vi "myRIO_BRig_FPGA_v3,61__PortC.vi"() -> ()   [LabVIEW 2014]
uses:
  <vilib>/rvi/Emulation/niFpgaGetClockAttributes.vi
  <vilib>/rvi/Emulation/niFpgaSctlEmulationGetInTimedLoop.vi
  <vilib>/rvi/Emulation/niFpgaEmulationReportErrorSimple.vi
  <vilib>/rvi/eio/common/nirviEmuTemplateMethod_errors.vi
  <vilib>/rvi/Emulation/niFpgaCriticalErrorInLSC.vi
  <vilib>/eio/EIONode/EIONode.xnode
panel:
  in  "laser2_selRew_Ntotal":u32=100
  in  "laser2selWro_Ntotal":u32=100
  in  "laser2_selRew_Ndelay":u32
  in  "laser2_selWro_Ndelay":u32
  in  "laser2_Npeak":u32=100
  in  "laser2_Nvalley":u32=100
  in  "laser2_Nshutter":u32=100
  in  "laser2_On":bool
  in  "laser2_Event":bool
  out "AnaIn_1":i16
  out "AnaIn_0":i16
  out "count_timeTrial":u32
  in  "timeTrial":bool
  in  "k1__counter_per_ms":u16=100 min=100 max=40000 step=1
  in  "laser1_Nshutter":u32=100
  in  "AnaOut_0":i16
  in  "laser1_Nvalley":u32=100
  in  "laser1_Npeak":u32=100
  in  "laser1_Event":bool
  in  "laser1_selWro_Ntotal":u32=100
  in  "laser1_selWro_Ndelay":u32
  in  "laser1_selRew_Ntotal":u32=100
  in  "laser1_selRew_Ndelay":u32
  in  "laserResponse_reward_LED":bool
  in  "laserResponse_wrong_LED":bool
  out "SelectWrong":bool
  out "SelectReward":bool
  in  "laserResponse_wrong":bool
  in  "laserResponse_reward":bool
  in  "Left(F)_or_Right(T)":bool
  in  "ignoreWrong":bool
  in  "SelectionState":bool
  in  "laser1_On":bool
  in  "FPGA_Stop":bool
  in  "audioTrigger_L":bool
  in  "audioTrigger_R":bool
  in  "audioFreq_L_kHz":u8=14 min=1 max=14 step=1
  in  "audioAmp_L":u16=1 min=1 max=32767 step=1
  in  "audioFreq_R_kHz":u8=14 min=1 max=14 step=1
  in  "audioAmp_R":u16=1 min=1 max=32767 step=1
  in  "A3_SL":bool
  in  "A1_SR":bool
  in  "Counts_Reset":bool
  out "A4_LickR":u32
  out "A2_LickL":u32
  in  "A6_Act":bool
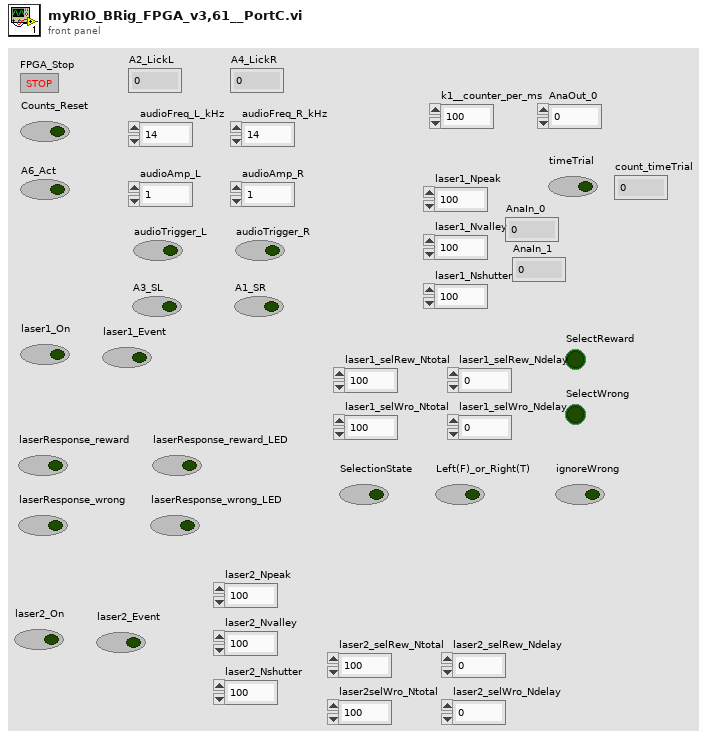
[diagram p1: front panel]
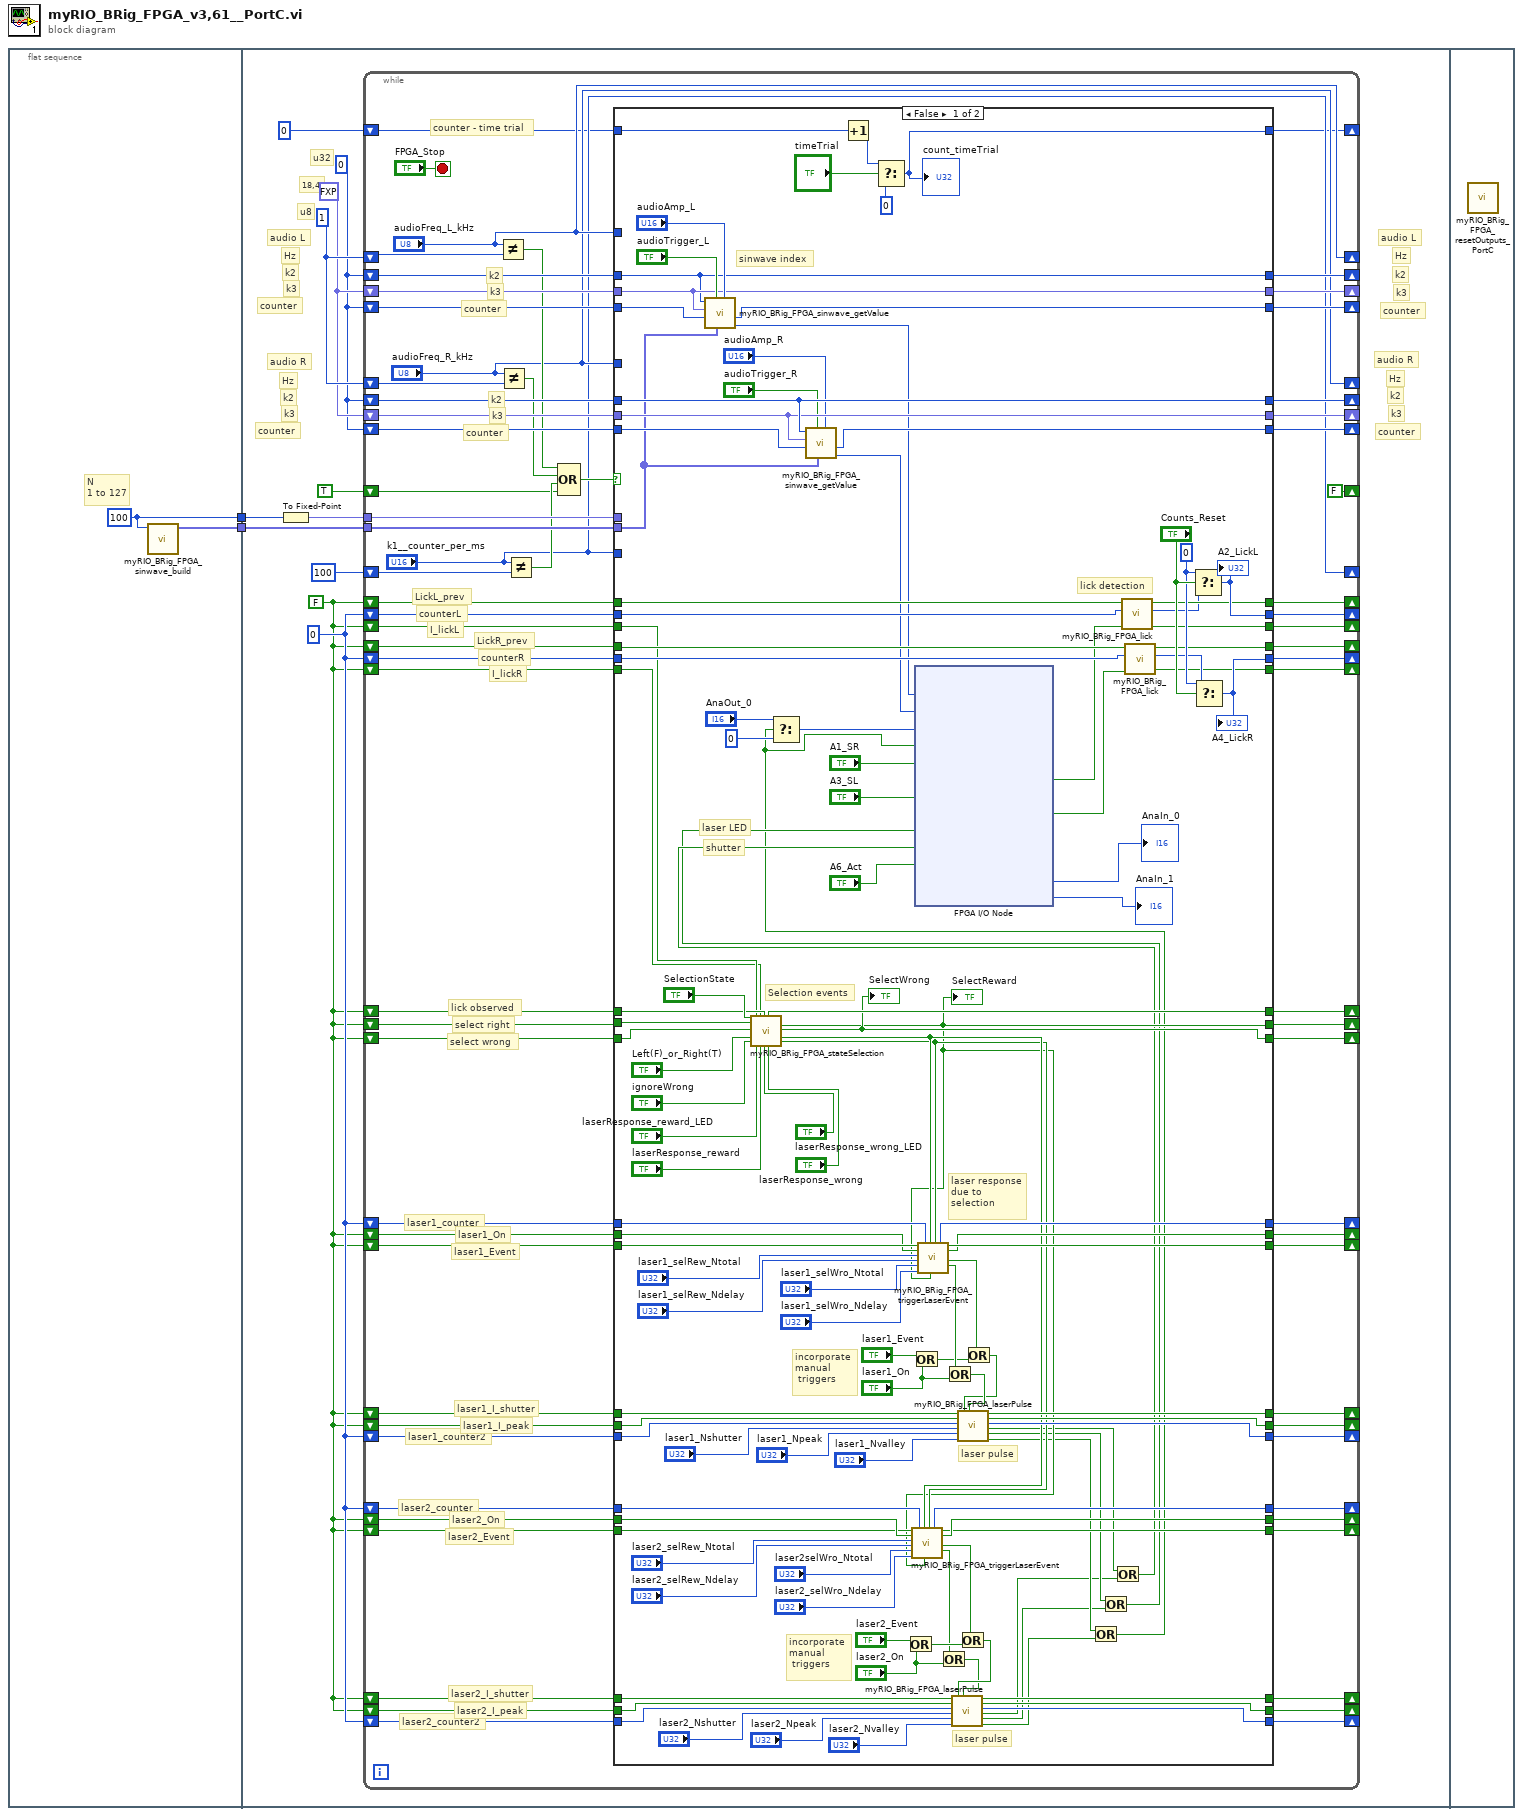
[diagram p0: block diagram]
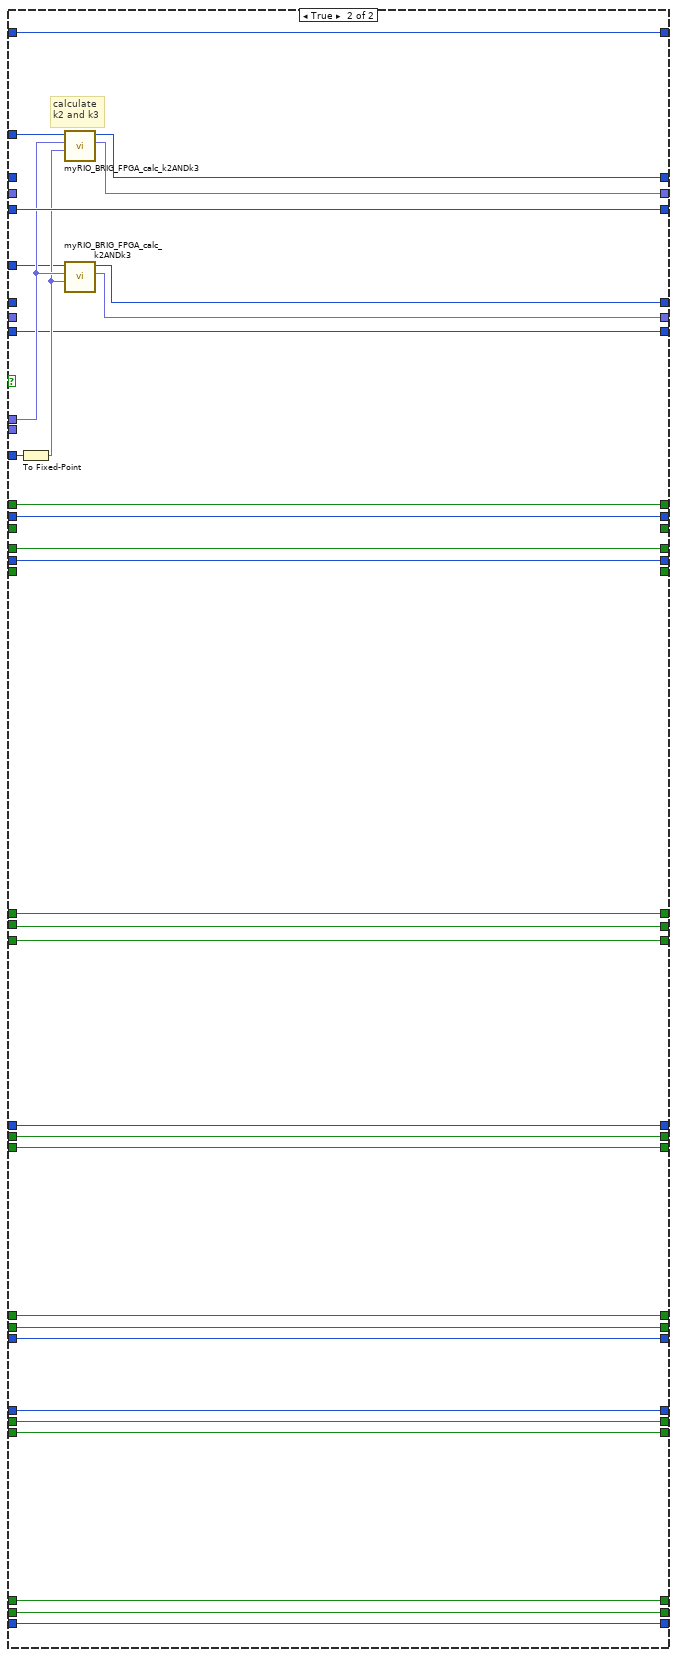
[diagram p2: hidden frame]
diagram:
  n1 = flat-sequence {
    tunnel: [w4] -> w2
    tunnel: [w3] -> w1
    tunnel: w2 -> [w15]
    tunnel: w1 -> [w14]
    frame #0 {
      w3 = 100 ("dimension size")
      # "N\n1 to 127"
      n2 = call "myRIO_BRig_FPGA_sinwave_build.vi"("input_Npts"=w3) -> ("output_array_sin"=w4:fxp<+/-,16,2>[])  [unwired: 10 in]
    }
    frame #1 {
      w6 = u32 0
      w5 = FALSE
      w10 = u32 0
      w11 = fxp<+,18,4> 0.0
      w12 = u8 1
      # "counter"
      # "k3"
      # "k2"
      # "counter"
      # "k3"
      # "k2"
      # "counter"
      # "counter"
      # "u32"
      # "k3"
      # "k2"
      # "k3"
      # "18,4"
      # "u8"
      # "Hz"
      # "Hz"
      # "audio R"
      # "audio L"
      # "Hz"
      # "k2"
      # "Hz"
      # "audio R"
      # "audio L"
      n3 = To Fixed-Point(number=w14) -> (fixed-point=w13:fxp<+,7,7>)  [unwired: 1 in]
      n4 = while {
        shift-right: ["audioFreq_L_kHz"] -> _
        shift-left: w12 -> [w86]
        shift-right: [w80] -> _
        shift-left: w10 -> [w84]
        shift-right: ["audioFreq_R_kHz"] -> _
        shift-left: w12 -> [w76]
        tunnel: w15 -> [w83]
        tunnel: w13 -> [w82]
        shift-right: [w79] -> _
        shift-left: w11 -> [w81]
        shift-right: [w77] -> _
        shift-left: w10 -> [w78]
        shift-right: [w74] -> _
        shift-left: w10 -> [w75]
        shift-right: [w72] -> _
        shift-left: w11 -> [w73]
        shift-right: [w70] -> _
        shift-left: w10 -> [w71]
        shift-right: ["k1__counter_per_ms"] -> _
        shift-left: u16 100 ("y") -> [w69]
        shift-right: [FALSE] -> _
        shift-left: TRUE -> [w64]
        shift-right: [w57] -> _
        shift-left: w5 -> [w59]
        shift-right: [w56] -> _
        shift-left: w5 -> [w58]
        shift-right: [w54] -> _
        shift-left: w6 -> [w55]
        shift-right: [w52] -> _
        shift-left: w6 -> [w53]
        shift-right: [w50] -> _
        shift-left: w5 -> [w51]
        shift-right: [w47] -> _
        shift-left: w5 -> [w49]
        shift-right: [w46] -> _
        shift-left: w5 -> [w48]
        shift-right: [w43] -> _
        shift-left: w5 -> [w42]
        shift-right: [w44] -> _
        shift-left: w5 -> [w45]
        shift-right: [w40] -> _
        shift-left: w6 -> [w41]
        shift-right: [w36] -> _
        shift-left: w5 -> [w39]
        shift-right: [w35] -> _
        shift-left: w5 -> [w38]
        shift-right: [w34] -> _
        shift-left: w6 -> [w37]
        shift-right: [w32] -> _
        shift-left: w5 -> [w33]
        shift-right: [w30] -> _
        shift-left: w5 -> [w31]
        shift-right: [w28] -> _
        shift-left: u32 0 -> [w29]
        shift-right: [w19] -> _
        shift-left: w5 -> [w23]
        shift-right: [w20] -> _
        shift-left: w5 -> [w22]
        shift-right: [w21] -> _
        shift-left: w6 -> [w24]
        shift-right: [w18] -> _
        shift-left: w5 -> [w25]
        shift-right: [w17] -> _
        shift-left: w5 -> [w26]
        shift-right: [w16] -> _
        shift-left: w6 -> [w27]
        stop <- "FPGA_Stop" stop-if-true
        # "laser2_counter2"
        # "laser2_counter"
        # "laser2_I_shutter"
        # "laser2_I_peak"
        # "laser2_On"
        # "laser2_Event"
        # "counter"
        # "k3"
        # "k2"
        # "counter"
        # "k3"
        # "k2"
        # "counter - time trial"
        # "laser1_counter2"
        # "laser1_counter"
        # "I_lickR"
        # "counterR"
        # "LickR_prev"
        # "I_lickL"
        # "counterL"
        # "LickL_prev"
        # "laser1_I_shutter"
        # "laser1_I_peak"
        # "laser1_On"
        # "laser1_Event"
        # "select wrong"
        # "select right"
        # "lick observed"
        n5 = Not Equal?(x="audioFreq_L_kHz", y=w86) -> (x != y?=w68:bool)
        n6 = Not Equal?(x="audioFreq_R_kHz", y=w76) -> (x != y?=w67:bool)
        n7 = Not Equal?(x="k1__counter_per_ms", y=w69) -> (x != y?=w65:bool)
        n8 = Compound Arithmetic op=OR(w68, w67, w65, w64) -> (w66:bool)
        n9 = case shown="False" w66 {
          tunnel: w84 -> [w174 _]
          tunnel: "audioFreq_L_kHz" -> [_ w238]
          tunnel: w83 -> [w167 _]
          tunnel: w82 -> [_ w234]
          tunnel: "k1__counter_per_ms" -> [_ w239]
          tunnel: w81 -> [w175 _]
          tunnel: [w174 w237] -> w80
          tunnel: [w175 w236] -> w79
          tunnel: w78 -> [w179 w235]
          tunnel: [w176 w235] -> w77
          tunnel: w75 -> [w171 _]
          tunnel: [w171 w230] -> w74
          tunnel: w73 -> [w170 _]
          tunnel: [w170 w231] -> w72
          tunnel: w71 -> [w173 w229]
          tunnel: "audioFreq_R_kHz" -> [_ w232]
          tunnel: [w172 w229] -> w70
          tunnel: w59 -> [w162 w228]
          tunnel: w58 -> [w161 w227]
          tunnel: [w166 w228] -> w57
          tunnel: [w159 w227] -> w56
          tunnel: w55 -> [w163 w226]
          tunnel: [w208 w226] -> w54
          tunnel: w53 -> [w160 w225]
          tunnel: [w205 w225] -> w52
          tunnel: w51 -> [w201 w224]
          tunnel: [w200 w224] -> w50
          tunnel: w49 -> [w203 w223]
          tunnel: w48 -> [w202 w222]
          tunnel: [w96 w223] -> w47
          tunnel: [w193 w222] -> w46
          tunnel: w45 -> [w191 w221]
          tunnel: [w187 w221] -> w44
          tunnel: [w188 w220] -> w43
          tunnel: w42 -> [w192 w220]
          tunnel: w41 -> [w190 w219]
          tunnel: [w189 w219] -> w40
          tunnel: w39 -> [w149 w218]
          tunnel: w38 -> [w150 w217]
          tunnel: w37 -> [w151 w216]
          tunnel: [w152 w218] -> w36
          tunnel: [w153 w217] -> w35
          tunnel: [w154 w216] -> w34
          tunnel: w33 -> [w156 _]
          tunnel: [w165 _] -> w32
          tunnel: w31 -> [w155 _]
          tunnel: [w157 _] -> w30
          tunnel: w29 -> [w139 w215]
          tunnel: [w136 w215] -> w28
          tunnel: w22 -> [w100 w213]
          tunnel: [w104 w213] -> w20
          tunnel: [w103 w212] -> w19
          tunnel: w23 -> [w99 w212]
          tunnel: w24 -> [w101 w214]
          tunnel: [w102 w214] -> w21
          tunnel: w25 -> [w115 w211]
          tunnel: w26 -> [w114 w210]
          tunnel: w27 -> [w113 w209]
          tunnel: [w112 w211] -> w18
          tunnel: [w111 w210] -> w17
          tunnel: [w110 w209] -> w16
          frame False {
            w206 = u32 0 ("t")
            # "laser pulse"
            # "incorporate\nmanual\n triggers"
            # "sinwave index"
            # "lick detection"
            # "laser pulse"
            # "incorporate\nmanual\n triggers"
            # "laser response\ndue to\nselection"
            # "Selection events"
            # "laser LED"
            # "shutter"
            n10 = call "myRIO_BRig_FPGA_sinwave_getValue.vi"("audioAmp"="audioAmp_L", "sinwave"=w167, "audioTrigger"="audioTrigger_L", "counter"=w179, "k3"=w175, "k2"=w174) -> ("output_audioValue"=w134:i16, "output_counter"=w176:u32)  [unwired: 4 in]
            n11 = call "myRIO_BRig_FPGA_stateSelection.vi"("I_selectionState"="SelectionState", "I_selectRight"=w203, "I_selectWrong"=w202, "I_Left(F)_or_Right(T)"="Left(F)_or_Right(T)", "I_ignoreWrong"="ignoreWrong", "I_lickL"=w156, "I_laserEvent_Reward"="laserResponse_reward_LED", "I_lickR"=w155, "I_laser_Reward"="laserResponse_reward", "I_lickObserved"=w201, "I_laserEvent_Wrong"="laserResponse_wrong_LED", "I_laser_Wrong"="laserResponse_wrong") -> ("output_I_lickObserved"=w200:bool, "output__I_selectRight"=w96:bool, "output__I_selectWrong"=w193:bool, "output_I_startLaserEvent"=w98:bool, "output_I_startLaser"=w97:bool)  [unwired: 11 in]
            "SelectWrong" <- w193
            "SelectReward" <- w96
            n12 = call "myRIO_BRig_FPGA_sinwave_getValue.vi"("audioAmp"="audioAmp_R", "sinwave"=w167, "audioTrigger"="audioTrigger_R", "counter"=w173, "k3"=w170, "k2"=w171) -> ("output_audioValue"=w133:i16, "output_counter"=w172:u32)  [unwired: 4 in]
            n13 = Increment(x=w139) -> (x+1=w138:u32)
            n14 = Select(t=w138, s="timeTrial", f=u32 0) -> (s? t:f=w136:u32)
            "count_timeTrial" <- w136
            n15 = Or(x="laser2_Event", y="laser2_On") -> (x .or. y?=w121:bool)
            n16 = Or(x="laser1_Event", y="laser1_On") -> (x .or. y?=w143:bool)
            n17 = call "myRIO_BRig_FPGA_triggerLaserEvent.vi"("I_laserEvent"=w99, "I_laser"=w100, "laser_selRew_Ntotal"="laser2_selRew_Ntotal", "laser_selRew_Ndelay"="laser2_selRew_Ndelay", "laser_selWro_Ntotal"="laser2selWro_Ntotal", "laser_selWro_NDelay"="laser2_selWro_Ndelay", "counter"=w101, "I_startLaserEvent"=w98, "selectReward"=w96, "I_startLaser"=w97) -> ("output_counter"=w102:u32, "output_I_laserEvent"=w103:bool, "output_I_laser"=w104:bool, "output_I_trigLaserEvent"=w119:bool, "output_I_trigLaser"=w120:bool)  [unwired: 5 in]
            n18 = call "myRIO_BRig_FPGA_triggerLaserEvent.vi"("I_laserEvent"=w192, "I_laser"=w191, "laser_selRew_Ntotal"="laser1_selRew_Ntotal", "laser_selRew_Ndelay"="laser1_selRew_Ndelay", "laser_selWro_Ntotal"="laser1_selWro_Ntotal", "laser_selWro_NDelay"="laser1_selWro_Ndelay", "counter"=w190, "I_startLaserEvent"=w98, "selectReward"=w96, "I_startLaser"=w97) -> ("output_counter"=w189:u32, "output_I_laserEvent"=w188:bool, "output_I_laser"=w187:bool, "output_I_trigLaserEvent"=w145:bool, "output_I_trigLaser"=w144:bool)  [unwired: 5 in]
            n19 = Or(x=w120, y="laser2_On") -> (x .or. y?=w123:bool)
            n20 = Or(x=w144, y="laser1_On") -> (x .or. y?=w141:bool)
            n21 = Or(x=w119, y=w121) -> (x .or. y?=w124:bool)
            n22 = call "myRIO_BRig_FPGA_laserPulse.vi"("I_shutter"=w115, "I_peak"=w114, "count"=w113, "laser_Nshutter"="laser2_Nshutter", "laser_Npeak"="laser2_Npeak", "laser_Nvalley"="laser2_Nvalley", "I_laserEvent"=w124, "I_laser"=w123) -> ("output_I_shutter"=w112:bool, "output_I_peak"=w111:bool, "output_count"=w110:u32, "output_shutter"=w89:bool, "output_led"=w88:bool, "output_laser"=w87:bool)  [unwired: 6 in]
            n23 = Or(x=w145, y=w143) -> (x .or. y?=w140:bool)
            n24 = call "myRIO_BRig_FPGA_laserPulse.vi"("I_shutter"=w149, "I_peak"=w150, "count"=w151, "laser_Nshutter"="laser1_Nshutter", "laser_Npeak"="laser1_Npeak", "laser_Nvalley"="laser1_Nvalley", "I_laserEvent"=w140, "I_laser"=w141) -> ("output_I_shutter"=w152:bool, "output_I_peak"=w153:bool, "output_count"=w154:u32, "output_shutter"=w95:bool, "output_led"=w94:bool, "output_laser"=w93:bool)  [unwired: 6 in]
            n25 = Or(x=w93, y=w87) -> (x .or. y?=w90:bool)
            n26 = Select(t="AnaOut_0", s=w90, f=i16 0) -> (s? t:f=w129:i16)
            n27 = Or(x=w94, y=w88) -> (x .or. y?=w91:bool)
            n28 = Or(x=w95, y=w89) -> (x .or. y?=w92:bool)
            n29 = xnode "FPGA I/O Node"("AudioOut/Left"=w134, "AudioOut/Right"=w133, "ConnectorC/AO0"=w129, "ConnectorC/DIO0"=w90, "ConnectorC/DIO1"="A1_SR", "ConnectorC/DIO3"="A3_SL", "ConnectorC/DIO5"=w91, "ConnectorC/DIO6"=w92, "ConnectorC/DIO7"="A6_Act") -> ("ConnectorC/DIO2"=w132:bool, "ConnectorC/DIO4"=w131:bool, "ConnectorC/AI0"=→"AnaIn_0":i16, "ConnectorC/AI1"=→"AnaIn_1":i16)  [unwired: 13 in, 13 out]
            n30 = call "myRIO_BRig_FPGA_lick.vi"("I_stateDetector_new"=w132, "counter"=w163, "I_stateDetector_prev"=w162) -> ("output_I_lick"=w165:bool, "output_counter"=w164:u32, "output_I_stateDetector_prev"=w166:bool)  [unwired: 6 in]
            n31 = call "myRIO_BRig_FPGA_lick.vi"("I_stateDetector_new"=w131, "counter"=w160, "I_stateDetector_prev"=w161) -> ("output_I_lick"=w157:bool, "output_counter"=w158:u32, "output_I_stateDetector_prev"=w159:bool)  [unwired: 6 in]
            n32 = Select(t=w206, s="Counts_Reset", f=w164) -> (s? t:f=w208:u32)
            "A2_LickL" <- w208
            n33 = Select(t=w206, s="Counts_Reset", f=w158) -> (s? t:f=w205:u32)
            "A4_LickR" <- w205
          }
          frame True {
            # "calculate\nk2 and k3"
            n34 = To Fixed-Point(number=w239) -> (fixed-point=w233:fxp<+,16,16>)  [unwired: 1 in]
            n35 = call "myRIO_BRIG_FPGA_calc_k2ANDk3.vi"("input_k1[count/ms]"=w233, "input_Npts"=w234, "input_freq[kHz]"=w238) -> ("output_k3"=w236:fxp<+,18,4>, "output_k2"=w237:u32)  [unwired: 7 in]
            n36 = call "myRIO_BRIG_FPGA_calc_k2ANDk3.vi"("input_k1[count/ms]"=w233, "input_Npts"=w234, "input_freq[kHz]"=w232) -> ("output_k3"=w231:fxp<+,18,4>, "output_k2"=w230:u32)  [unwired: 7 in]
          }
        }
      }
    }
    frame #2 {
      n37 = call "myRIO_BRig_FPGA_resetOutputs_PortC.vi"() -> ()  [unwired: 12 in]
    }
  }
